vi "428_READER1.vi"(8 "error in (no error)":errorcluster, 10 "Command 1":string, 11 "VISA resource name":refnum<visa-resource-name>) -> (0 "error out":errorcluster, 2 "Wavelength":string="0000.0000\r\n", 3 "VISA resource name out":refnum<visa-resource-name>)   [LabVIEW 2016]
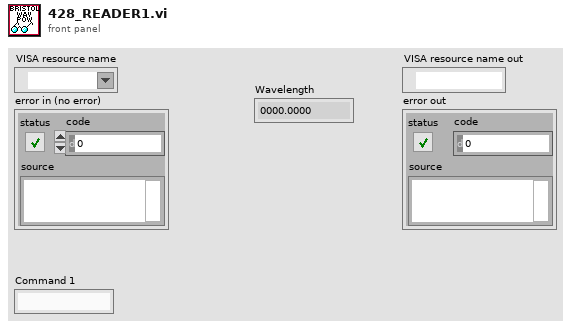
[diagram p1: front panel]
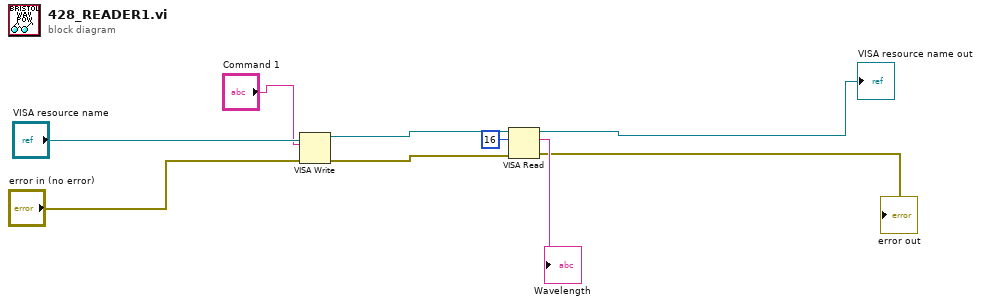
[diagram p0: block diagram]
diagram:
  n1 = VISA Write(VISA resource name="VISA resource name", write buffer="Command 1", error in (no error)="error in (no error)") -> (VISA resource name out=w9:refnum<visa-resource-name>, error out=w8:errorcluster)  [unwired: 1 out]
  n2 = VISA Read(VISA resource name=w9, byte count=u32 16, error in (no error)=w8) -> (VISA resource name out=→"VISA resource name out":refnum<visa-resource-name>, read buffer=→"Wavelength":string, error out=→"error out":errorcluster)  [unwired: 1 out]
